vi "Bit Time Parameter.vi"(0 "section":string, 11 "Error in":errorcluster) -> (4 "This VI":refnum<vi>, 15 "Error out":errorcluster)   [LabVIEW 2020, in "Speed Mode.lvclass"]
uses:
  Speed Mode.lvclass
  <vilib>/Utility/config.llb/Read Key (Double).vi
  <vilib>/Utility/config.llb/NI_LVConfig.lvlib
panel:
  in  "Time Parameter":T1
  in  "T buf":dbl format="%#_g µs"
  in  "T high":dbl format="%#_g µs"
  in  "T low":dbl format="%#_g µs"
  in  "T hd:dat":dbl format="%#_g µs"
  in  "T su:dat":dbl format="%#_g ns"
  in  "T su:sto":dbl format="%#_g µs"
  in  "T hd:sta":dbl format="%#_g µs"
  in  "T su:sta":dbl format="%#_g µs"
  in  "Clock Frequency":dbl format="%#_g kHz"
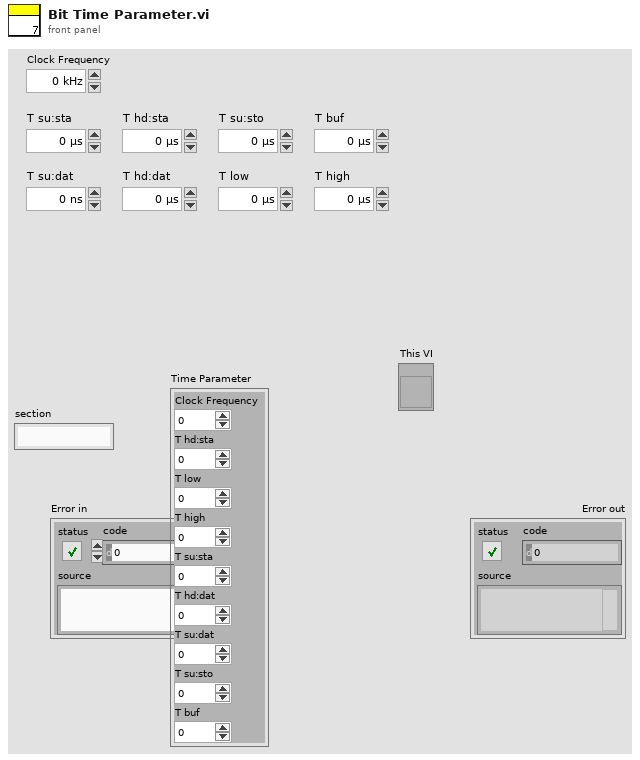
[diagram p1: front panel]
types:
  T1 = cluster{"Clock Frequency":dbl, "T hd:sta":dbl, "T low":dbl, "T high":dbl, "T su:sta":dbl, "T hd:dat":dbl, "T su:dat":dbl, "T su:sto":dbl, "T buf":dbl}
  T2 = typedef "NI_LVConfig.lvlib/Config Data RefNum.ctl" = refnum<k1>
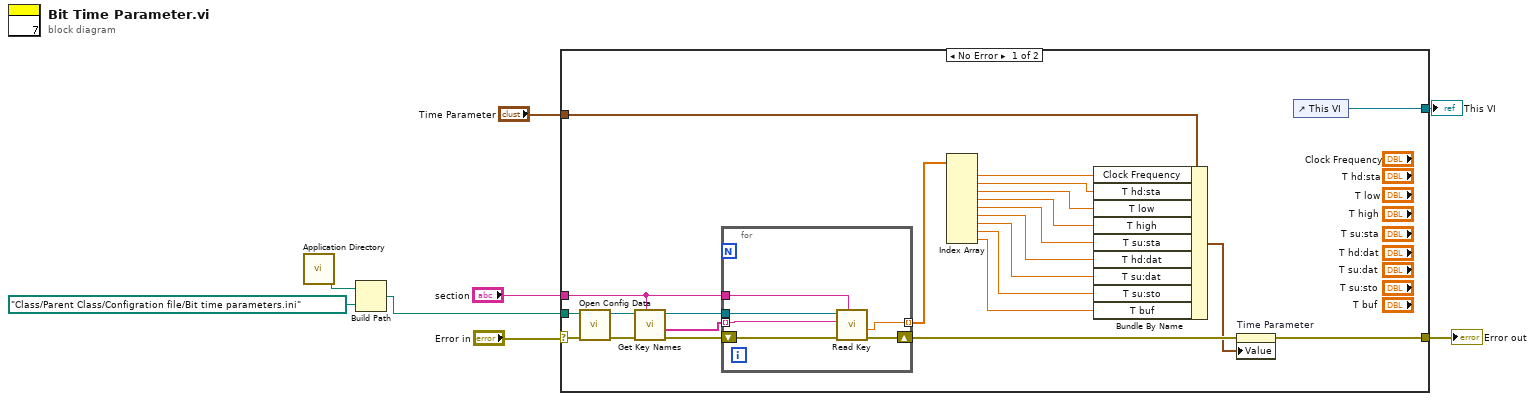
[diagram p0: block diagram]
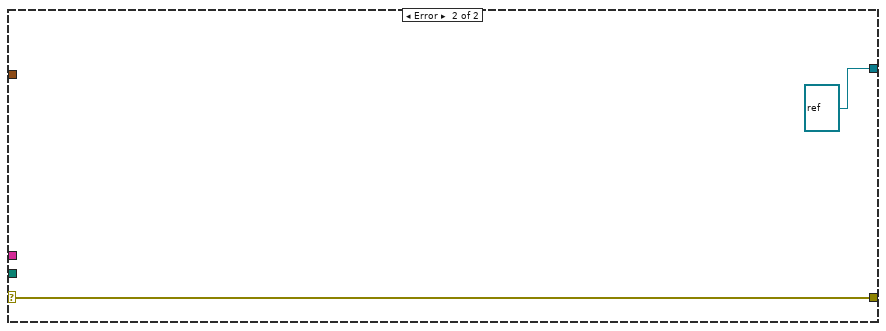
[diagram p2: hidden frame]
diagram:
  n1 = call <vilib>:"Application Directory.vi"() -> ("Application Directory"=w8:path)
  n2 = Build Path(base path=w8, name or relative path=path "Class/Parent Class/Configration file/Bit time parameters.ini") -> (appended path=w3:path)
  n3 = case shown="No Error" "Error in" {
    selector: "Error in" -> [w29 w39]
    tunnel: [w20 w39] -> w5
    tunnel: "section" -> [w25 _]
    tunnel: w3 -> [w22 _]
    tunnel: [w21 refnum<vi> refnum ("This VI")] -> w2
    tunnel: "Time Parameter" -> [w19 _]
    frame No Error {
      n4 = call <vilib>:"Open Config Data.vi"("error in (no error)"=w29, "configuration file path"=w22) -> ("error out"=w31:errorcluster, "refnum"=w30:T2)  [unwired: 7 in, 1 out]
      n5 = call <vilib>:"Get Key Names.vi"("section"=w25, "error in (no error)"=w31, "refnum"=w30) -> ("error out"=w28:errorcluster, "key names"=w24:string[], "refnum out"=w26:T2)  [unwired: 5 in, 1 out]
      n6 = for {
        tunnel: w26 -> [w35]
        tunnel: w25 -> [w34]
        shift-right: [w36] -> w27
        shift-left: w28 -> [w37]
        tunnel: w24 -> [w33] mode=indexing
        tunnel: [w32] -> w23 mode=indexing
        n7 = call-poly <vilib>:"Read Key.vi"("section"=w34, "error in (no error)"=w37, "key"=w33, "refnum"=w35) -> ("error out"=w36:errorcluster, "value"=w32:dbl)  [unwired: 4 in, 2 out]
      }
      n8 = Index Array(array=w23) -> (element #1=w18:dbl, element #2=w16:dbl, element #3=w15:dbl, element #4=w14:dbl, element #5=w13:dbl, element #6=w12:dbl, element #7=w11:dbl, element #8=w10:dbl, element #9=w9:dbl)  [unwired: 9 in]
      n9 = Bundle By Name(cluster=w19, "Clock Frequency"=w18, "T hd:sta"=w16, "T low"=w15, "T high"=w14, "T su:sta"=w13, "T hd:dat"=w12, "T su:dat"=w11, "T su:sto"=w10, "T buf"=w9) -> (w17:T1)
      n10 = property on="Time Parameter" class="Clust (strict)"(error in=w27, "Value"=w17) -> (error out=w20:errorcluster)  [unwired: 1 in, 1 out]
      n11 = control-ref of="This VI"() -> (w21:refnum<vi>)
    }
    frame Error {
    }
  }
  "Error out" <- w5
  "This VI" <- w2
